vi "inbuild_smtp_send_mail.vi"() -> ()   [LabVIEW 2014]
uses:
  <vilib>/smtpClient/Set Message Text.vi
  <vilib>/smtpClient/LabVIEWSMTPClient.lvlib
panel:
  in  "body of the message":string
  in  "subject":string
  in  "password":string
  in  "username":string
  in  "from":string
  in  "to":string[](array[string])
  in  "port":string
  in  "mail smtp":string
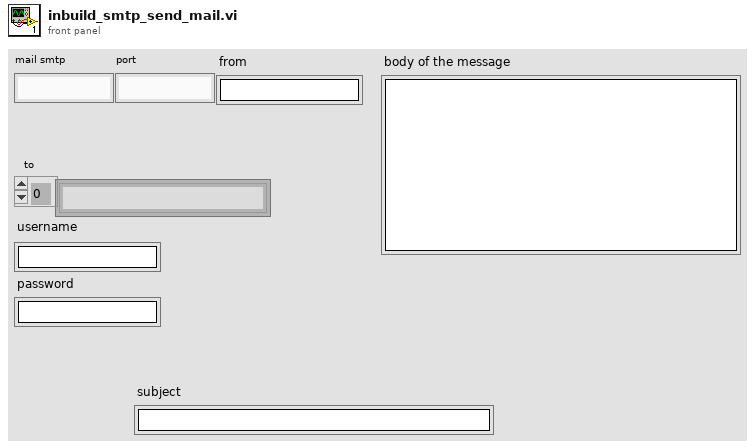
[diagram p1: front panel]
types:
  T1 = typedef "LabVIEWSMTPClient.lvlib/SmtpClientHandle.ctl" = refnum<k1>
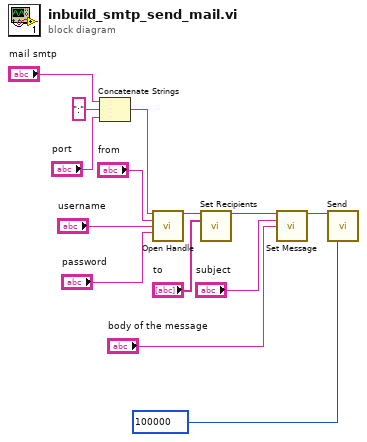
[diagram p0: block diagram]
diagram:
  n1 = Concatenate Strings("mail smtp", ":" ("string"), "port") -> (w12:string)
  n2 = call <vilib>:"Open Handle.vi"("server address"=w12, "from"="from", "username"="username", "password"="password") -> ("handle out"=w11:T1)  [unwired: 10 in, 1 out]
  n3 = call <vilib>:"Set Recipients.vi"("handle in"=w11, "to"="to") -> ("handle out"=w14:T1)  [unwired: 12 in, 1 out]
  n4 = call-poly <vilib>:"Set Message.vi"("handle in"=w14, "subject"="subject", "plain text message"="body of the message") -> ("handle out"=w13:T1)  [unwired: 11 in, 1 out]
  n5 = call <vilib>:"Send.vi"("handle in"=w13, "timeout in ms (10000)"=100000) -> ()  [unwired: 11 in, 3 out]
